vi "AIT 1553 - ReadWrite LoopStats.vi"(5 "Late":bool, 6 "Iteration Duration":i64, 7 "Mode":T1, 8 "error in (no error)":errorcluster, 11 "RT Data in":T2 {"Acyclic Frame Refs" format="%.0x"; "Label Transfer Config"."Block Data Refs"."Data Reference" format="%.0x"; "Status Config"."HWOut Dur Ref" format="%.0x"; "Status Config"."HWIn Dur Ref" format="%.0x"; "Status Config"."HWOut Count Ref" format="%.0x"; "Status Config"."HWIn Count Ref" format="%.0x"; "Status Config"."Error Data Ref" format="%.0x"; "HWOutput Channels"."Message Settings"."Driver Data"."First Word" min=8 max=31; "HWOutput Channels"."Message Settings"."Driver Data"."Num Bits" min=1 max=32; "HWOutput Channels"."Message Settings"."Driver Data"."Start Bit" min=8 max=31; "HWOutput Channels"."Message Settings"."Block Data Refs"."Data Reference" format="%.0x"; "HWInput Channels"."Message Settings"."Driver Data"."First Word" min=8 max=31; "HWInput Channels"."Message Settings"."Driver Data"."Num Bits" min=1 max=32; "HWInput Channels"."Message Settings"."Driver Data"."Start Bit" min=8 max=31; "HWInput Channels"."Message Settings"."Block Data Refs"."Data Reference" format="%.0x"}) -> (0 "error out":errorcluster, 3 "RT Data out":T2 {"Acyclic Frame Refs" format="%.0x"; "Label Transfer Config"."Block Data Refs"."Data Reference" format="%.0x"; "Status Config"."HWOut Dur Ref" format="%.0x"; "Status Config"."HWIn Dur Ref" format="%.0x"; "Status Config"."HWOut Count Ref" format="%.0x"; "Status Config"."HWIn Count Ref" format="%.0x"; "Status Config"."Error Data Ref" format="%.0x"; "HWOutput Channels"."Message Settings"."Driver Data"."First Word" min=8 max=31; "HWOutput Channels"."Message Settings"."Driver Data"."Num Bits" min=1 max=32; "HWOutput Channels"."Message Settings"."Driver Data"."Start Bit" min=8 max=31; "HWOutput Channels"."Message Settings"."Block Data Refs"."Data Reference" format="%.0x"; "HWInput Channels"."Message Settings"."Driver Data"."First Word" min=8 max=31; "HWInput Channels"."Message Settings"."Driver Data"."Num Bits" min=1 max=32; "HWInput Channels"."Message Settings"."Driver Data"."Start Bit" min=8 max=31; "HWInput Channels"."Message Settings"."Block Data Refs"."Data Reference" format="%.0x"})   [LabVIEW 2013, in "AIT 1553 Custom Device.lvlib"]
uses:
  AIT 1553 Custom Device.lvlib
  RT Controls/AIT 1553  - RT Data.ctl
  RT Controls/AIT 1553 - RT HW Channel.ctl
  RT Controls/AIT 1553 - Bus Section.ctl
  RT Controls/AIT 1553 - RT Message Settings.ctl
  <vilib>/NI Veristand/Custom Device API/Block Data Reference.ctl
  <vilib>/NI Veristand/Custom Device API/Data Reference.ctl
  RT Controls/AIT 1553 - Driver Data.ctl
  Controls and Global/Start Bit.ctl
  Controls and Global/Number of Bits.ctl
  RT Controls/AIT 1553 - Board Config Info.ctl
  RT Controls/AIT 1553 - Hardware Type.ctl
  RT Controls/Error Qs.ctl
  RT Controls/Status Channels Config.ctl
  RT Controls/FIFO.ctl
  RT Controls/Label Transfer Config.ctl
  <vilib>/NI Veristand/Custom Device API/Custom Device Item Ref.ctl
  RT Controls/ReadWrite Selector.ctl
  <vilib>/NI Veristand/Custom Device API/Global Data Refs.vi
  <vilib>/NI Veristand/Custom Device API/Custom Device API.lvlib
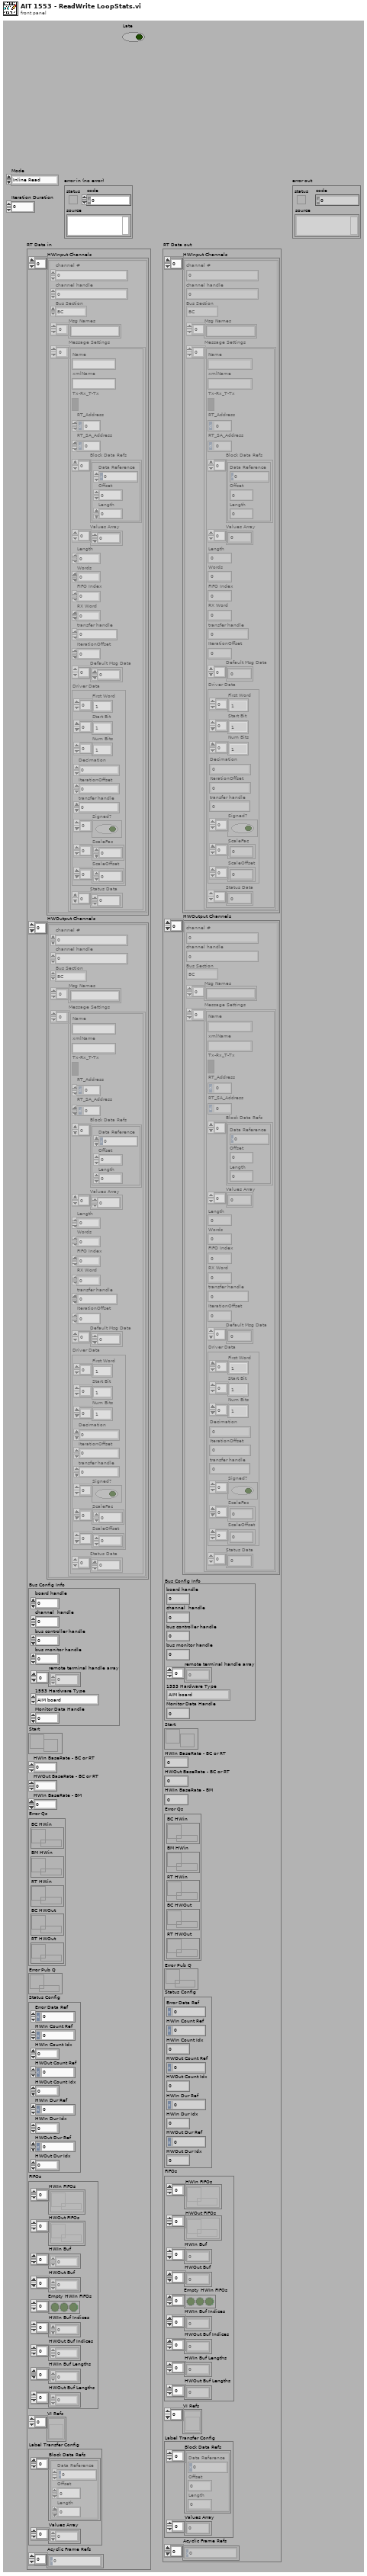
[diagram p1: front panel]
types:
  T1 = typedef "AIT 1553 Custom Device.lvlib/ReadWrite Selector.ctl" = enum16{"Inline Read", "Inline Write", "Async HWIn", "Async HWOut"}
  T2 = typedef "AIT 1553 Custom Device.lvlib/AIT 1553  - RT Data.ctl" = cluster{"HWInput Channels":T3[], "HWOutput Channels":T3[], "Bus Config Info":T11, "Start":refnum<notifier>, "HWIn BaseRate - BC or RT":i64, "HWOut BaseRate - BC or RT":i64, "HWIn BaseRate - BM":i64, "Error Qs":T13, "Error Pub Q":refnum<queue>, "Status Config":T14, "FIFOs":T15, "VI Refs":refnum<vi>[], "Label Transfer Config":T16, "Acyclic Frame Refs":T17[]}
  T3 = typedef "AIT 1553 Custom Device.lvlib/AIT 1553 - RT HW Channel.ctl" = cluster{"channel #":u16, "channel handle":u32, "Bus Section":T4, "Msg Names":string[], "Message Settings":T5[]}
  T4 = typedef "AIT 1553 Custom Device.lvlib/AIT 1553 - Bus Section.ctl" = enum16{"BC", "BM", "RT"}
  T5 = typedef "AIT 1553 Custom Device.lvlib/AIT 1553 - RT Message Settings.ctl" = cluster{"Name":string, "xmlName":string, "Tx-Rx_T-Tx":bool, "RT_Address":u8, "RT_SA_Address":u8, "Block Data Refs":T6[], "Values Array":dbl[], "Length":i32, "Words":i32, "FIFO Index":i32, "RX Word":u32, "transfer handle":u32, "IterationOffset":i32, "Default Msg Data":u16[], "Driver Data":T8, "Status Data":u32[]}
  T6 = typedef "Custom Device API.lvlib/Block Data Reference.ctl" = cluster{"Data Reference":T7, "Offset":i32, "Length":i32}
  T7 = typedef "Custom Device API.lvlib/Data Reference.ctl" = i32
  T8 = typedef "AIT 1553 Custom Device.lvlib/AIT 1553 - Driver Data.ctl" = cluster{"First Word":T9[], "Start Bit":T9[], "Num Bits":T10[], "Decimation":i32, "IterationOffset":i32, "transfer handle":u32, "Signed?":bool[], "ScaleFac":dbl[], "ScaleOffset":dbl[]}
  T9 = typedef "AIT 1553 Custom Device.lvlib/Start Bit.ctl" = i32
  T10 = typedef "AIT 1553 Custom Device.lvlib/Number of Bits.ctl" = i32
  T11 = typedef "AIT 1553 Custom Device.lvlib/AIT 1553 - Board Config Info.ctl" = cluster{"board handle":u32, "channel  handle":u32, "bus controller handle":u32, "bus monitor handle":u32, "remote terminal handle array":u32[], "1553 Hardware Type":T12, "Monitor Data Handle":u32}
  T12 = typedef "AIT 1553 Custom Device.lvlib/AIT 1553 - Hardware Type.ctl" = enum16{"AIM board", "AIT Board"}
  T13 = typedef "AIT 1553 Custom Device.lvlib/Error Qs.ctl" = cluster{"BC HWin":refnum<queue>, "BM HWin":refnum<queue>, "RT HWin":refnum<queue>, "BC HWOut":refnum<queue>, "RT HWOut":refnum<queue>}
  T14 = typedef "AIT 1553 Custom Device.lvlib/Status Channels Config.ctl" = cluster{"Error Data Ref":T7, "HWIn Count Ref":T7, "HWIn Count Idx":i32, "HWOut Count Ref":T7, "HWOut Count Idx":i32, "HWIn Dur Ref":T7, "HWIn Dur Idx":i32, "HWOut Dur Ref":T7, "HWOut Dur Idx":i32}
  T15 = typedef "AIT 1553 Custom Device.lvlib/FIFO.ctl" = cluster{"HWIn FIFOs":refnum<k33>[], "HWOut FIFOs":refnum<k33>[], "HWIn Buf":dbl[], "HWOut Buf":dbl[], "Empty HWIn FIFOs":bool[], "HWIn Buf Indices":i32[], "HWOut Buf Indices":i32[], "HWIn Buf Lengths":i32[], "HWOut Buf Lengths":i32[]}
  T16 = typedef "AIT 1553 Custom Device.lvlib/Label Transfer Config.ctl" = cluster{"Block Data Refs":T6[], "Values Array":dbl[]}
  T17 = typedef "Custom Device API.lvlib/Custom Device Item Ref.ctl" = u64
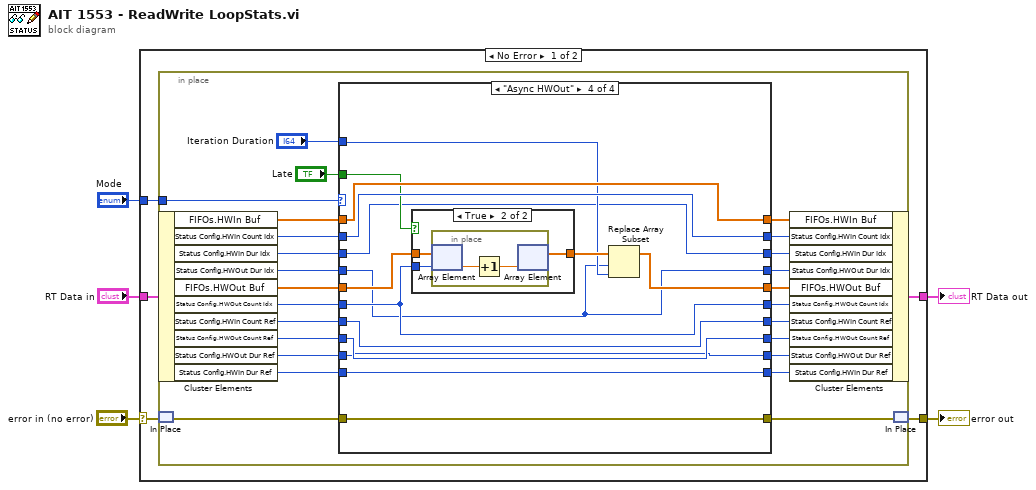
[diagram p0: block diagram]
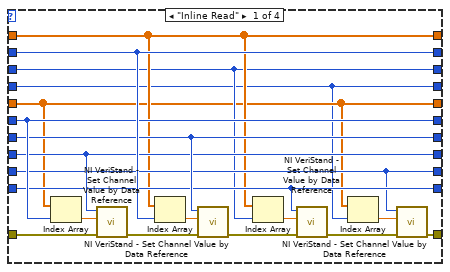
[diagram p2: hidden frame]
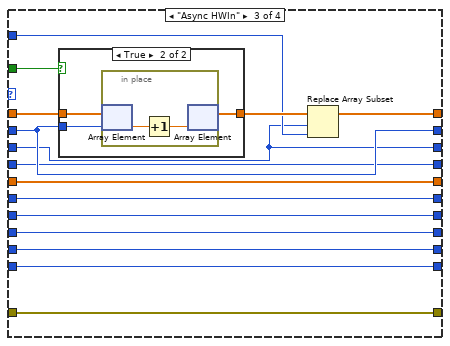
[diagram p4: hidden frame]
diagram:
  n1 = case shown="No Error" "error in (no error)" {
    selector: "error in (no error)" -> [w9 w109]
    tunnel: "RT Data in" -> [w10 w108]
    tunnel: [w8 w108] -> w3
    tunnel: [w7 w109] -> w2
    tunnel: "Mode" -> [w6 _]
    frame No Error {
      n2 = in-place {
        in-place-border: w6 -> [w27]
        n3 = in-place-cluster #1(w10) -> ("FIFOs.HWIn Buf"=w35:dbl[], "Status Config.HWIn Count Idx"=w34:i32, "Status Config.HWIn Dur Idx"=w23:i32, "Status Config.HWOut Dur Idx"=w21:i32, "FIFOs.HWOut Buf"=w33:dbl[], "Status Config.HWOut Count Idx"=w32:i32, "Status Config.HWIn Count Ref"=w29:T7, "Status Config.HWOut Count Ref"=w28:T7, "Status Config.HWOut Dur Ref"=w20:T7, "Status Config.HWIn Dur Ref"=w19:T7)
        n4 = in-place-match #2(w9) -> (w31:errorcluster)
        n5 = case shown="\"Async HWOut\"" w27 {
          tunnel: w35 -> [w41 w59 w74 w98]
          tunnel: w34 -> [w50 w60 w73 w97]
          tunnel: w33 -> [w37 w61 w80 w95]
          tunnel: w32 -> [w49 w62 w79 w94]
          tunnel: w31 -> [w54 w65 w76 w99]
          tunnel: [w45 w65 w76 w99] -> w30
          tunnel: w29 -> [w48 w63 w77 w100]
          tunnel: w28 -> [w47 w64 w78 w101]
          tunnel: [w47 w64 w78 w101] -> w15
          tunnel: [w48 w63 w77 w100] -> w14
          tunnel: [w49 w62 w79 w94] -> w26
          tunnel: [w37 w61 w80 w92] -> w25
          tunnel: [w50 w60 w73 w97] -> w11
          tunnel: [w41 w59 w71 w98] -> w18
          tunnel: "Late" -> [_ _ w75 w96]
          tunnel: w23 -> [w39 w57 w69 w90]
          tunnel: "Iteration Duration" -> [_ _ w70 w91]
          tunnel: [w39 w57 w69 w90] -> w12
          tunnel: [w36 w58 w68 w89] -> w13
          tunnel: w21 -> [w36 w58 w68 w89]
          tunnel: [w42 w56 w67 w88] -> w16
          tunnel: w20 -> [w42 w56 w67 w88]
          tunnel: [w43 w55 w66 w87] -> w17
          tunnel: w19 -> [w43 w55 w66 w87]
          frame "Inline Read" {
            n6 = Index Array(array=w37, index=w49) -> (element=w52:dbl)
            n7 = call <vilib>:"NI VeriStand - Set Channel Value by Data Reference.vi"("error in (no error)"=w54, "Value"=w52, "Data Reference in"=w47) -> ("error out"=w51:errorcluster)  [unwired: 8 in]
            n8 = Index Array(array=w41, index=w50) -> (element=w53:dbl)
            n9 = call <vilib>:"NI VeriStand - Set Channel Value by Data Reference.vi"("error in (no error)"=w51, "Value"=w53, "Data Reference in"=w48) -> ("error out"=w46:errorcluster)  [unwired: 8 in]
            n10 = Index Array(array=w41, index=w39) -> (element=w40:dbl)
            n11 = call <vilib>:"NI VeriStand - Set Channel Value by Data Reference.vi"("error in (no error)"=w46, "Value"=w40, "Data Reference in"=w43) -> ("error out"=w44:errorcluster)  [unwired: 8 in]
            n12 = Index Array(array=w37, index=w36) -> (element=w38:dbl)
            n13 = call <vilib>:"NI VeriStand - Set Channel Value by Data Reference.vi"("error in (no error)"=w44, "Value"=w38, "Data Reference in"=w42) -> ("error out"=w45:errorcluster)  [unwired: 8 in]
          }
          frame Default {
          }
          frame "Async HWIn" {
            n14 = case shown="True" w75 {
              tunnel: w74 -> [w81 w84]
              tunnel: w73 -> [_ w83]
              tunnel: [w81 w82] -> w72
              frame False {
              }
              frame True {
                n15 = in-place {
                  n16 = in-place-array #3(w84, w83) -> (w86:dbl)
                  n17 = Increment(x=w86) -> (x+1=w85:dbl)
                  n18 = in-place-array #3(w85) -> (w82:dbl[])  [unwired: 1 out]
                }
              }
            }
            n19 = Replace Array Subset(array=w72, new element=w70, index=w69) -> (w71:dbl[])
          }
          frame "Async HWOut" {
            n20 = case shown="True" w96 {
              tunnel: [w102 w105] -> w93
              tunnel: w95 -> [w102 w104]
              tunnel: w94 -> [_ w103]
              frame False {
              }
              frame True {
                n21 = in-place {
                  n22 = in-place-array #4(w104, w103) -> (w107:dbl)
                  n23 = Increment(x=w107) -> (x+1=w106:dbl)
                  n24 = in-place-array #4(w106) -> (w105:dbl[])  [unwired: 1 out]
                }
              }
            }
            n25 = Replace Array Subset(array=w93, new element=w91, index=w89) -> (w92:dbl[])
          }
        }
        n26 = in-place-cluster #1("FIFOs.HWIn Buf"=w18, "Status Config.HWIn Count Idx"=w11, "Status Config.HWIn Dur Idx"=w12, "Status Config.HWOut Dur Idx"=w13, "FIFOs.HWOut Buf"=w25, "Status Config.HWOut Count Idx"=w26, "Status Config.HWIn Count Ref"=w14, "Status Config.HWOut Count Ref"=w15, "Status Config.HWOut Dur Ref"=w16, "Status Config.HWIn Dur Ref"=w17) -> (w8:T2)
        n27 = in-place-match #2(w30) -> (w7:errorcluster)
      }
    }
    frame Error {
    }
  }
  "error out" <- w2
  "RT Data out" <- w3
